vi "热敏电阻温度转换子程序.vi"(9 "U":dbl, 10 "Vcc":dbl=5.0, 11 "R":dbl=10.0) -> (1 "Rt":dbl, 2 "t":dbl)   [LabVIEW 2015]
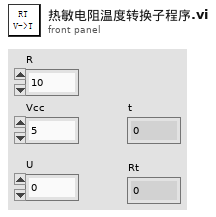
[diagram p1: front panel]
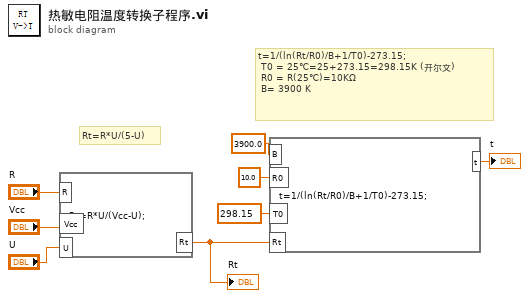
[diagram p0: block diagram]
diagram:
  # "t=1/(ln(Rt/R0)/B+1/T0)-273.15;\n T0 = 25℃=25+273.15=298.15K (开尔文)\n R0 = R(25℃)=10KΩ\n B= 3900 K"
  # "Rt=R*U/(5-U)"
  n1 = formula code="Rt=R*U/(Vcc-U);"("U"="U", "R"="R", "Vcc"="Vcc") -> ("Rt"=w5:dbl)
  "Rt" <- w5
  n2 = formula code="t=1/(ln(Rt/R0)/B+1/T0)-273.15;"("Rt"=w5, "B"=3900.0 ("B值"), "R0"=10.0, "T0"=298.15) -> ("t"=→"t":dbl)
